vi "GT Set Pre Vltg.vi"(7 "channel":i16, 8 "error in (no error)":errorcluster caption="错误输入（无错误）", 9 "voltageValue":dbl, 10 "mode":u16, 11 "cardNum":i16) -> (0 "error out":errorcluster caption="错误输出", 3 "function return":i16)   [LabVIEW 2014, in "gts.lvlib"]
doc: "GT_API GT_SetPreVltg(short cardNum,unsigned short mode,double voltageValue,short channel=0);"
uses:
  gts.lvlib
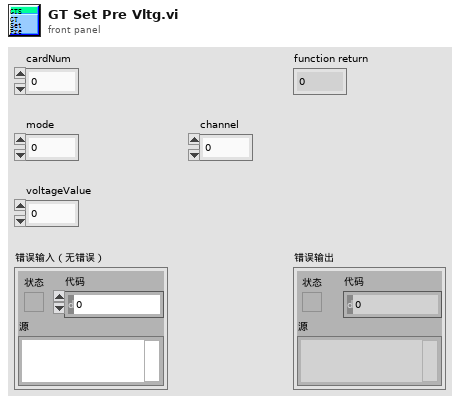
[diagram p1: front panel]
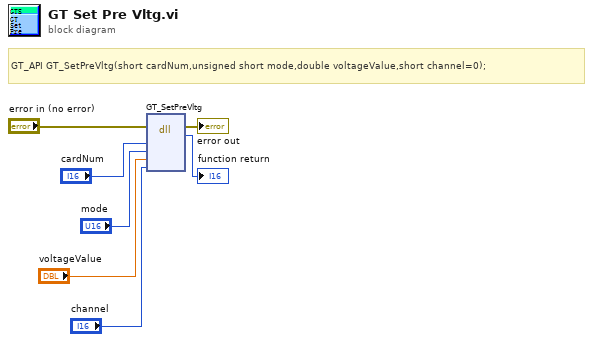
[diagram p0: block diagram]
diagram:
  # "GT_API GT_SetPreVltg(short cardNum,unsigned short mode,double voltageValue,short channel=0);"
  n1 = dll-call lib="PTH2habs D固高科技资料GTS控制卡GTS卡18年上半年资料dllVC32bit\nmulti_cardgts.*" fn="GT_SetPreVltg"(error in="error in (no error)", "cardNum"="cardNum", "mode"="mode", "voltageValue"="voltageValue", "channel"="channel") -> (error out=→"error out":errorcluster, →"function return":i16)  [unwired: 6 in, 1 out]
